vi "post.vi"(8 "error in (no error)":errorcluster, 10 "build_spec":T1, 11 "lv-build-default in":refnum<class "lv-builder-default.lvclass">) -> (0 "error out":errorcluster, 3 "lv-build-default out":refnum<class "lv-builder-default.lvclass">)   [LabVIEW 2015, in "lv-builder-default.lvclass"]
uses:
  lv-builder-default.lvclass
  lv-build/public/_controls/build_specification.ctl
  lv-build/public/_controls/build_type.ctl
  _controls/configuration.ctl
  _controls/post_action_lvlib.ctl
  _controls/post_action_zip.ctl
  _controls/post_action_application.ctl
  _controls/post_action_installer.ctl
  lv-builder/public/accessors/project_file_read.vi
  lv-builder-default.lvlib
  lv-build/lv-build.lvlib
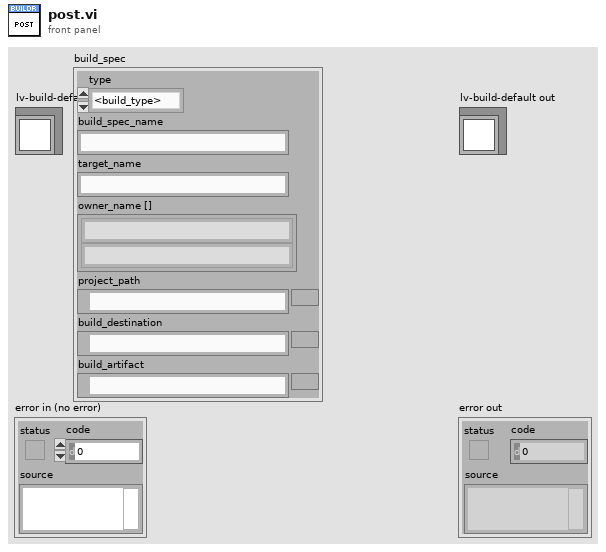
[diagram p1: front panel]
types:
  T1 = typedef "lv-build.lvlib/build_specification.ctl" = cluster{"type":T2, "build_spec_name":string, "target_name":string, "owner_name []":string[], "project_path":path, "build_destination":path, "build_artifact":path}
  T2 = typedef "lv-build.lvlib/build_type.ctl" = enum16{"<build_type>", "application_pc", "application_rt", "installer", "llb", "lvlibp", "zip", "fpga", "<null>"}
  T3 = typedef "lv-builder-default.lvlib/configuration.ctl" = cluster{"project_file":string, "lvlibp_directory":string, "zip_directory":string, "lvlib_directory":string, "update_version_vi":string, "installer_post_file":string, "distribution_folder":string, "dependencies_folder":string, "version":string, "bin_folder":string, "lvlib_post_action":u16, "installer_post_action":u16, "application_post_action":u16, "zip_post_action":u16}
  T4 = typedef "lv-builder-default.lvlib/post_action_lvlib.ctl" = enum16{"<lvlib_post_action>", "nothing", "move", "install", "<null>"}
  T5 = typedef "lv-builder-default.lvlib/post_action_zip.ctl" = enum16{"<zip_post_action>", "nothing", "move", "extract", "<null>"}
  T6 = typedef "lv-builder-default.lvlib/post_action_application.ctl" = enum16{"<application_post_action>", "nothing", "zip_application", "<null>"}
  T7 = typedef "lv-builder-default.lvlib/post_action_installer.ctl" = enum16{"<installer_post_action>", "nothing", "create_installer", "zip_installer", "create_installer_file", "<null>"}
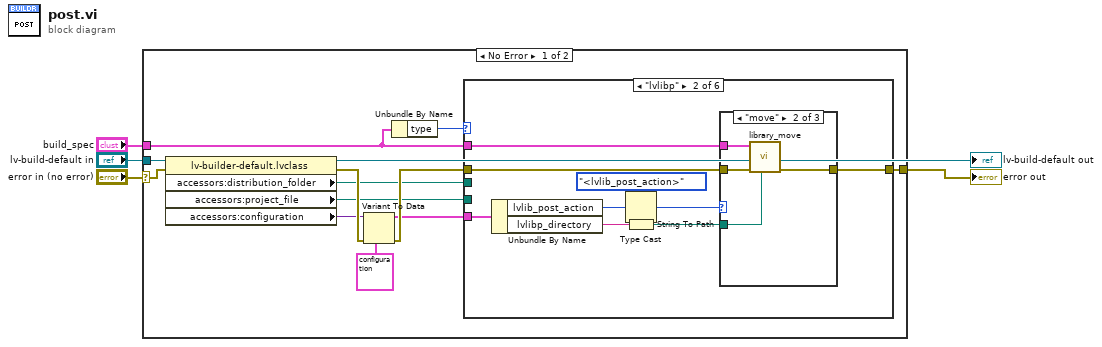
[diagram p0: block diagram]
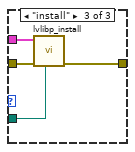
[diagram p4: hidden frame]
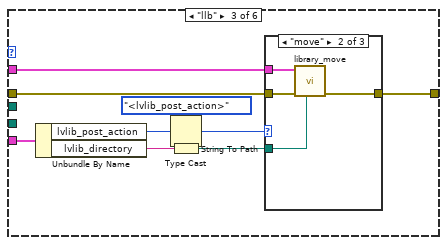
[diagram p5: hidden frame]
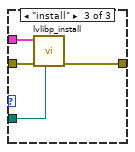
[diagram p7: hidden frame]
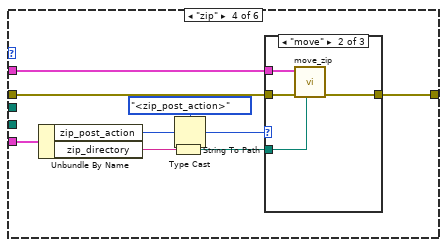
[diagram p8: hidden frame]
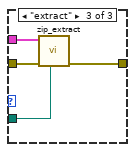
[diagram p10: hidden frame]
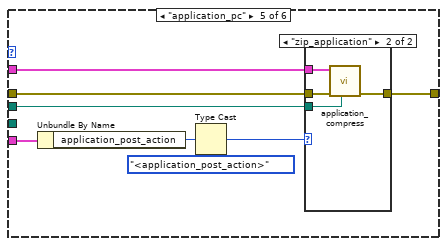
[diagram p11: hidden frame]
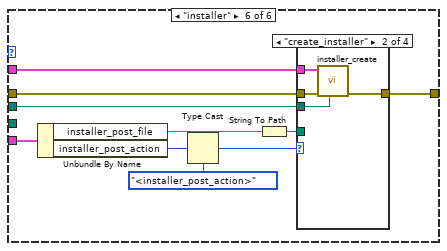
[diagram p13: hidden frame]
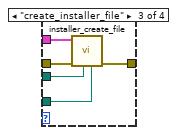
[diagram p15: hidden frame]
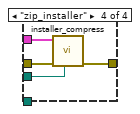
[diagram p16: hidden frame]
diagram:
  n1 = case shown="No Error" "error in (no error)" {
    selector: "error in (no error)" -> [w12 w109]
    tunnel: [w15 w109] -> w4
    tunnel: "build_spec" -> [w14 _]
    tunnel: "lv-build-default in" -> [w11 _]
    frame No Error {
      n2 = property class="lv-builder-default.lvclass"(reference=w11, error in=w12) -> (error out=w8:errorcluster, "accessors:distribution_folder"=w6:path, "accessors:project_file"=w5:path, "accessors:configuration"=w7:variant)  [unwired: 1 out]
      n3 = Variant To Data(error in=w8, type=T3 {"project_file"="", "lvlibp_directory"="", "zip_directory"="", "lvlib_directory"="", "update_version_vi"="", "installer_post_file"="", "distribution_folder"="", "dependencies_folder"="", "version"="", "bin_folder"="", "lvlib_post_action"=0, "installer_post_action"=0, "application_post_action"=0, "zip_post_action"=0} ("configuration"), Variant=w7) -> (data=w9:T3, error out=w16:errorcluster)
      n4 = Unbundle By Name(w14) -> ("type"=w13:T2)
      n5 = case shown="\"lvlibp\"" w13 {
        tunnel: [w17 w26 w44 w62 w79 w94] -> w15
        tunnel: w14 -> [_ w25 w43 w61 w78 w93]
        tunnel: w16 -> [w17 w24 w42 w60 w77 w92]
        tunnel: w6 -> [_ _ _ _ w72 w85]
        tunnel: w9 -> [_ w20 w38 w56 w73 w90]
        tunnel: w5 -> [_ _ _ _ _ _]
        frame Default {
        }
        frame "lvlibp" {
          n6 = Unbundle By Name(w20) -> ("lvlib_post_action"=w22:u16, "lvlibp_directory"=w19:string)
          n7 = Type Cast(type=post_action_lvlib."<lvlib_post_action>" ("lvlib_post_action"), x=w22) -> (*(type *) &x=w21:T4)
          n8 = String To Path(string=w19) -> (path=w18:path)
          n9 = case shown="\"move\"" w21 {
            tunnel: [w27 w29 w33] -> w26
            tunnel: w25 -> [_ w30 w35]
            tunnel: w24 -> [w27 w31 w34]
            tunnel: w18 -> [_ w28 w32]
            frame Default {
            }
            frame "move" {
              n10 = call "library_move.vi"("lvlib_move_directory"=w28, "error in (no error)"=w31, "build_specifications"=w30) -> ("error out"=w29:errorcluster)  [unwired: 8 in]
            }
            frame "install" {
              n11 = call "lvlibp_install.vi"("lvlib_move_directory"=w32, "error in (no error)"=w34, "build_specifications"=w35) -> ("error out"=w33:errorcluster)  [unwired: 8 in]
            }
          }
        }
        frame "llb" {
          n12 = Unbundle By Name(w38) -> ("lvlib_post_action"=w40:u16, "lvlib_directory"=w37:string)
          n13 = Type Cast(type=post_action_lvlib."<lvlib_post_action>" ("lvlib_post_action"), x=w40) -> (*(type *) &x=w39:T4)
          n14 = String To Path(string=w37) -> (path=w36:path)
          n15 = case shown="\"move\"" w39 {
            tunnel: [w45 w47 w51] -> w44
            tunnel: w43 -> [_ w48 w53]
            tunnel: w42 -> [w45 w49 w52]
            tunnel: w36 -> [_ w46 w50]
            frame Default {
            }
            frame "move" {
              n16 = call "library_move.vi"("lvlib_move_directory"=w46, "error in (no error)"=w49, "build_specifications"=w48) -> ("error out"=w47:errorcluster)  [unwired: 8 in]
            }
            frame "install" {
              n17 = call "lvlibp_install.vi"("lvlib_move_directory"=w50, "error in (no error)"=w52, "build_specifications"=w53) -> ("error out"=w51:errorcluster)  [unwired: 8 in]
            }
          }
        }
        frame "zip" {
          n18 = Unbundle By Name(w56) -> ("zip_post_action"=w59:u16, "zip_directory"=w55:string)
          n19 = String To Path(string=w55) -> (path=w54:path)
          n20 = Type Cast(type=post_action_zip."<zip_post_action>" ("zip_post_action"), x=w59) -> (*(type *) &x=w58:T5)
          n21 = case shown="\"move\"" w58 {
            tunnel: [w63 w65 w69] -> w62
            tunnel: w61 -> [_ w66 w70]
            tunnel: w60 -> [w63 w67 w71]
            tunnel: w54 -> [_ w64 w68]
            frame Default {
            }
            frame "move" {
              n22 = call "move_zip.vi"("zip_move_directory"=w64, "error in (no error)"=w67, "build_specifications"=w66) -> ("error out"=w65:errorcluster)  [unwired: 8 in]
            }
            frame "extract" {
              n23 = call "zip_extract.vi"("zip_extract_directory"=w68, "error in (no error)"=w71, "build_specifications"=w70) -> ("error out"=w69:errorcluster)  [unwired: 8 in]
            }
          }
        }
        frame "application_pc" {
          n24 = Unbundle By Name(w73) -> ("application_post_action"=w75:u16)
          n25 = Type Cast(type=post_action_application."<application_post_action>" ("application_post_action"), x=w75) -> (*(type *) &x=w74:T6)
          n26 = case shown="\"zip_application\"" w74 {
            tunnel: [w80 w82] -> w79
            tunnel: w78 -> [_ w84]
            tunnel: w77 -> [w80 w83]
            tunnel: w72 -> [_ w81]
            frame "nothing", Default {
            }
            frame "zip_application" {
              n27 = call "application_compress.vi"("distribution_folder"=w81, "error in (no error)"=w83, "build_specifications"=w84) -> ("error out"=w82:errorcluster)  [unwired: 8 in]
            }
          }
        }
        frame "installer" {
          n28 = Unbundle By Name(w90) -> ("installer_post_file"=w86:string, "installer_post_action"=w87:u16)
          n29 = Type Cast(type=post_action_installer."<installer_post_action>" ("installer_post_action"), x=w87) -> (*(type *) &x=w88:T7)
          n30 = String To Path(string=w86) -> (path=w91:path)
          n31 = case shown="\"create_installer\"" w88 {
            tunnel: [w95 w97 w102 w106] -> w94
            tunnel: w93 -> [_ w98 w103 w108]
            tunnel: w92 -> [w95 w99 w104 w107]
            tunnel: w91 -> [_ _ w100 _]
            tunnel: w85 -> [_ w96 w101 w105]
            frame "nothing", Default {
            }
            frame "create_installer" {
              n32 = call "installer_create.vi"("distribution_folder"=w96, "error in (no error)"=w99, "build_specifications"=w98) -> ("error out"=w97:errorcluster)  [unwired: 8 in]
            }
            frame "create_installer_file" {
              n33 = call "installer_create_file.vi"("special_file"=w100, "distribution_folder"=w101, "error in (no error)"=w104, "build_specifications"=w103) -> ("error out"=w102:errorcluster)  [unwired: 7 in]
            }
            frame "zip_installer" {
              n34 = call "installer_compress.vi"("distribution_folder"=w105, "error in (no error)"=w107, "build_specifications"=w108) -> ("error out"=w106:errorcluster)  [unwired: 8 in]
            }
          }
        }
      }
    }
    frame Error {
    }
  }
  "error out" <- w4
  "lv-build-default out" <- "lv-build-default in"
